vi "Objects to GUIDs.vi"(3 "error in (no error)":errorcluster, 4 "Objects":refnum<class "ObjectSettings.lvclass">[](array[class])) -> (0 "error out":errorcluster, 1 "GUIDs":string[](array[string]))   [LabVIEW 2019, in "Setting Database.lvclass"]
uses:
  Setting Database.lvclass
  ObjectSettings/ObjectSettings.lvclass
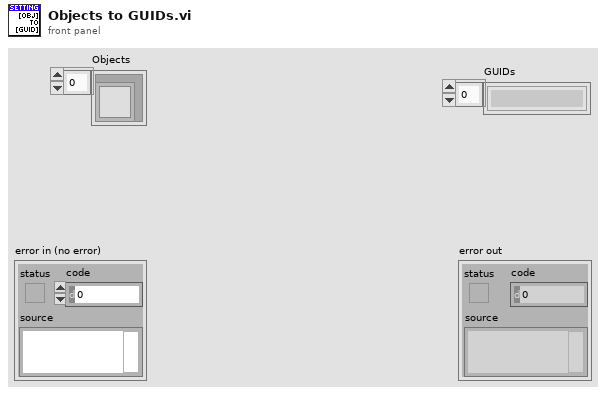
[diagram p1: front panel]
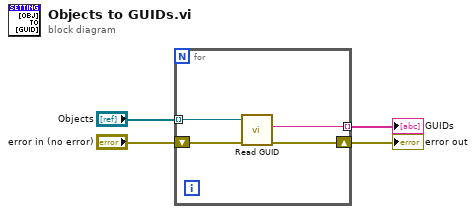
[diagram p0: block diagram]
diagram:
  n1 = for {
    tunnel: "Objects" -> [w8] mode=indexing
    tunnel: [w7] -> w3 mode=indexing
    shift-right: [w5] -> w1
    shift-left: "error in (no error)" -> [w6]
    n2 = call-dynamic "Read GUID.vi"("error in (no error)"=w6, "ObjectSettings in"=w8) -> ("error out"=w5:errorcluster, "GUID"=w7:string)  [unwired: 7 in, 1 out]
  }
  "error out" <- w1
  "GUIDs" <- w3
